vi "AxB.vi"(1 "B":dbl[](array[numeric]), 2 "A":dbl[](array[numeric])) -> (0 "AxB":dbl[](array[numeric]))   [LabVIEW 2011]
panel:
  # "="
  # "x"
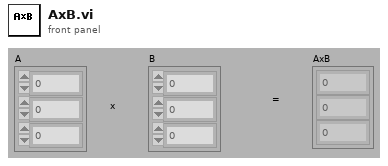
[diagram p1: front panel]
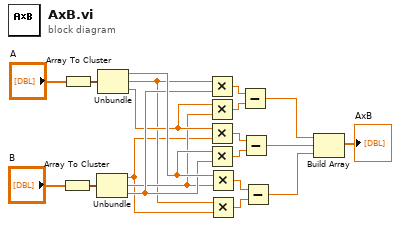
[diagram p0: block diagram]
diagram:
  n1 = Array To Cluster(array="B") -> (cluster=w13:cluster{"B[0]":dbl, "B[1]":dbl, "B[2]":dbl})
  n2 = Array To Cluster(array="A") -> (cluster=w15:cluster{"A[0]":dbl, "A[1]":dbl, "A[2]":dbl})
  n3 = Unbundle(w13) -> ("B[0]"=w1:dbl, "B[1]"=w5:dbl, "B[2]"=w8:dbl)
  n4 = Unbundle(w15) -> ("A[0]"=w9:dbl, "A[1]"=w2:dbl, "A[2]"=w6:dbl)
  n5 = Multiply(x=w2, y=w8) -> (x*y=w10:dbl)
  n6 = Multiply(x=w6, y=w5) -> (x*y=w12:dbl)
  n7 = Multiply(x=w6, y=w1) -> (x*y=w11:dbl)
  n8 = Multiply(x=w9, y=w8) -> (x*y=w7:dbl)
  n9 = Multiply(x=w9, y=w5) -> (x*y=w4:dbl)
  n10 = Multiply(x=w2, y=w1) -> (x*y=w3:dbl)
  n11 = Subtract(x=w10, y=w12) -> (x-y=w18:dbl)
  n12 = Subtract(x=w11, y=w7) -> (x-y=w19:dbl)
  n13 = Subtract(x=w4, y=w3) -> (x-y=w20:dbl)
  n14 = Build Array(w18, w19, w20) -> (→"AxB":dbl[])
